vi "HttpPut.vi"(6 "request specific headers":T1[](array[typedef]), 7 "binary string":bool, 8 "error in":errorcluster, 9 "body":string, 10 "url":string, 11 "reQwestClient in":refnum<class "reQwestClient.lvclass">) -> (0 "error out":errorcluster, 2 "response_body":string, 3 "reQwestClient out":refnum<class "reQwestClient.lvclass">)   [LabVIEW 2020, in "reQwestClient.lvclass"]
uses:
  reQwestClient.lvclass
  <vilib>/addons/_JKI.lib/REST Client/classes/REST Client/HTTP Header.ctl
  submodules/reqwest-rs-labview/lv_src/Types/http_method_enum.ctl
  reQwestClient.lvclass/reQwestClient.ctl
  submodules/reqwest-rs-labview/lv_src/Request/Request.lvclass
  submodules/reqwest-rs-labview/lv_src/Client/Client.lvclass
  submodules/reqwest-rs-labview/lv_src/reqwest.lvlib
  submodules/reqwest-rs-labview/lv_src/RequestBuilder/RequestBuilder.lvclass
  submodules/reqwest-rs-labview/lv_src/Headers/Headers.lvclass
  <vilib>/addons/_JKI.lib/REST Client/classes/REST Client/REST Client.lvclass
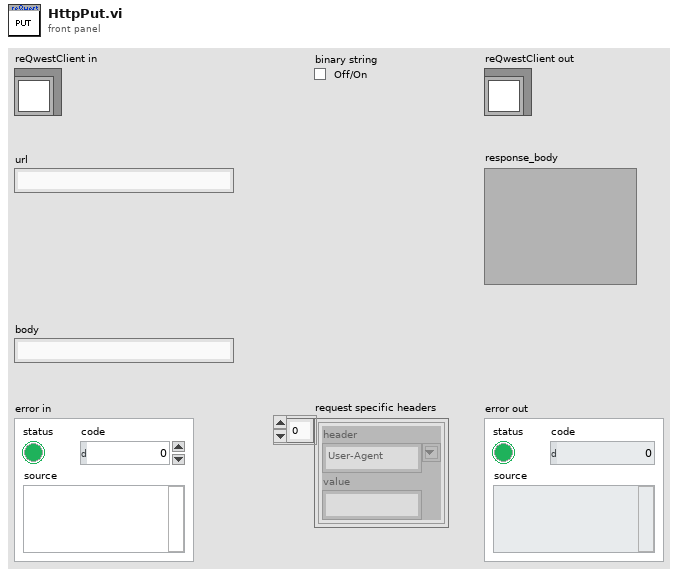
[diagram p1: front panel]
types:
  T1 = typedef "REST Client.lvlib/REST Client.lvclass/HTTP Header.ctl" = cluster{"header":string, "value":string}
  T2 = typedef "reqwest.lvlib/http_method_enum.ctl" = enum8{"<select>", "GET", "POST", "PUT", "DELETE", "HEAD", "OPTIONS", "CONNECT", "PATCH", "TRACE"}
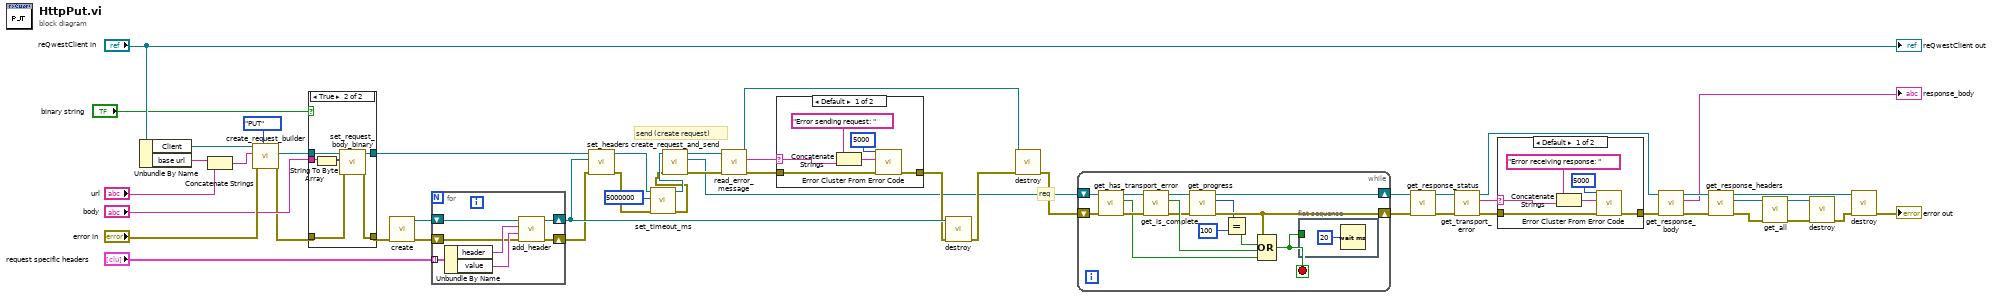
[diagram p0: block diagram]
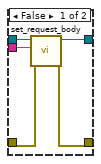
[diagram p2: hidden frame]
diagram:
  # "send (create request)"
  # "req"
  n1 = Unbundle By Name("reQwestClient in") -> ("Client"=w32:refnum<class "Client.lvclass">, "base url"=w22:string)
  n2 = Concatenate Strings(w22, "url") -> (w20:string)
  n3 = call "create_request_builder.vi"("HTTP Method"=http_method_enum."PUT", "error in (no error)"="error in", "url"=w20, "Client in"=w32) -> ("error out"=w9:errorcluster, "RequestBuilder out"=w12:refnum<class "RequestBuilder.lvclass">)  [unwired: 5 in, 1 out]
  n4 = case shown="True" "binary string" {
    tunnel: w12 -> [w55 w61]
    tunnel: "body" -> [w54 w57]
    tunnel: [w53 w60] -> w10
    tunnel: w9 -> [w52 w59]
    tunnel: [w51 w58] -> w8
    frame False {
      n5 = call "set_request_body.vi"("error in"=w52, "body"=w54, "obj in"=w55) -> ("error out"=w51:errorcluster, "obj out"=w53:refnum<class "RequestBuilder.lvclass">)  [unwired: 6 in, 1 out]
    }
    frame True {
      n6 = String To Byte Array(string=w57) -> (unsigned byte array=w56:u8[])
      n7 = call "set_request_body_binary.vi"("error in"=w59, "binary body"=w56, "obj in"=w61) -> ("error out"=w58:errorcluster, "obj out"=w60:refnum<class "RequestBuilder.lvclass">)  [unwired: 6 in, 1 out]
    }
  }
  n8 = call "create.vi"("error in (no error)"=w8) -> ("error out"=w29:errorcluster, "Headers out"=w31:refnum<class "Headers.lvclass">)  [unwired: 9 in]
  n9 = for {
    tunnel: "request specific headers" -> [w67] mode=indexing
    shift-right: [w63] -> w28
    shift-left: w31 -> [w68]
    shift-right: [w62] -> w26
    shift-left: w29 -> [w64]
    n10 = Unbundle By Name(w67) -> ("header"=w66:string, "value"=w65:string)
    n11 = call "add_header.vi"("error in (no error)"=w64, "value"=w65, "key"=w66, "Headers in"=w68) -> ("error out"=w62:errorcluster, "Headers out"=w63:refnum<class "Headers.lvclass">)  [unwired: 5 in, 1 out]
  }
  n12 = call "set_headers.vi"("error in (no error)"=w26, "Headers"=w28, "obj in"=w10) -> ("error out"=w4:errorcluster, "obj out"=w5:refnum<class "RequestBuilder.lvclass">)  [unwired: 6 in, 1 out]
  n13 = call "set_timeout_ms.vi"("error in (no error)"=w4, "timeout_ms"=u64 5000000, "obj in"=w5) -> ("error out"=w1:errorcluster, "obj out"=w2:refnum<class "RequestBuilder.lvclass">)  [unwired: 6 in, 1 out]
  n14 = call "create_request_and_send.vi"("error in"=w1, "obj in"=w2) -> ("error out"=w35:errorcluster, "request"=w6:refnum<class "Request.lvclass">, "obj out"=w36:refnum<class "RequestBuilder.lvclass">)  [unwired: 7 in]
  n15 = call "read_error_message.vi"("error in (no error)"=w35, "RequestBuilder in"=w36) -> ("error out"=w19:errorcluster, "error_message"=w17:string, "RequestBuilder in"=w37:refnum<class "RequestBuilder.lvclass">)  [unwired: 7 in]
  n16 = case shown="Default" w17 {
    selector: w17 -> [w71 _]
    tunnel: w19 -> [w74 w75]
    tunnel: [w73 w75] -> w18
    frame Default {
      n17 = Concatenate Strings("Error sending request: " ("error message (\"\")"), w71) -> (w72:string)
      n18 = call <vilib>:"Error Cluster From Error Code.vi"("error in (no error)"=w74, "error message (\"\")"=w72, "error code (0)"=5000) -> ("error out"=w73:errorcluster)  [unwired: 6 in]
    }
    frame "" {
    }
  }
  n19 = call "destroy.vi"("error in (no error)"=w18, "Headers in"=w28) -> ("error out"=w27:errorcluster)  [unwired: 9 in]
  n20 = call "destroy.vi"("error in"=w27, "RequestBuilder in"=w37) -> ("error out"=w34:errorcluster)  [unwired: 8 in, 1 out]
  n21 = while {
    shift-right: [w87] -> w41
    shift-left: w6 -> [w80]
    shift-right: [w85] -> w40
    shift-left: w34 -> [w79]
    stop <- w81 stop-if-true
    n22 = call "get_has_transport_error.vi"("error in (no error)"=w79, "Request in"=w80) -> ("error out"=w77:errorcluster, "has_transport_error"=w76:bool, "Request out"=w78:refnum<class "Request.lvclass">)  [unwired: 7 in]
    n23 = call "get_is_complete.vi"("error in (no error)"=w77, "Request in"=w78) -> ("error out"=w86:errorcluster, "is_complete"=w89:bool, "Request out"=w88:refnum<class "Request.lvclass">)  [unwired: 7 in]
    n24 = call "get_progress.vi"("error in (no error)"=w86, "Request in"=w88) -> ("error out"=w85:errorcluster, "progress"=w83:i32, "Request out"=w87:refnum<class "Request.lvclass">)  [unwired: 7 in]
    n25 = Equal?(x=w83, y=100 ("progress")) -> (x = y?=w82:bool)
    n26 = Compound Arithmetic op=OR(w85, w82, w89, w76) -> (w81:bool)
    n27 = flat-sequence {
      tunnel: w81 -> [_]
      frame #0 {
        n28 = Wait (ms)(milliseconds to wait=u32 20) -> ()  [unwired: 1 out]
      }
    }
  }
  n29 = call "get_response_status.vi"("error in (no error)"=w40, "Request in"=w41) -> ("error out"=w39:errorcluster, "Request out"=w38:refnum<class "Request.lvclass">)  [unwired: 7 in, 1 out]
  n30 = call "get_transport_error.vi"("error in (no error)"=w39, "Request in"=w38) -> ("error out"=w15:errorcluster, "transport_error"=w16:string, "Request in"=w13:refnum<class "Request.lvclass">)  [unwired: 7 in]
  n31 = case shown="Default" w16 {
    selector: w16 -> [w93 _]
    tunnel: w15 -> [w96 w97]
    tunnel: [w95 w97] -> w14
    frame Default {
      n32 = Concatenate Strings("Error receiving response: " ("error message (\"\")"), w93) -> (w94:string)
      n33 = call <vilib>:"Error Cluster From Error Code.vi"("error in (no error)"=w96, "error message (\"\")"=w94, "error code (0)"=5000) -> ("error out"=w95:errorcluster)  [unwired: 6 in]
    }
    frame "" {
    }
  }
  n34 = call "get_response_body.vi"("error in (no error)"=w14, "Request in"=w13) -> ("error out"=w47:errorcluster, "string_value"=→"response_body":string, "Request in"=w49:refnum<class "Request.lvclass">)  [unwired: 7 in]
  n35 = call "get_response_headers.vi"("error in (no error)"=w47, "Request in"=w49) -> ("error out"=w45:errorcluster, "response_headers"=w46:refnum<class "Headers.lvclass">, "Request in"=w48:refnum<class "Request.lvclass">)  [unwired: 7 in]
  n36 = call "get_all.vi"("error in (no error)"=w45, "Headers in"=w46) -> ("error out"=w43:errorcluster, "Headers in"=w44:refnum<class "Headers.lvclass">)  [unwired: 6 in, 2 out]
  n37 = call "destroy.vi"("error in (no error)"=w43, "Headers in"=w44) -> ("error out"=w42:errorcluster)  [unwired: 9 in]
  n38 = call "destroy.vi"("error in (no error)"=w42, "Request in"=w48) -> ("error out"=→"error out":errorcluster)  [unwired: 8 in, 1 out]
  "reQwestClient out" <- "reQwestClient in"
